vi "V-Meter Shutdown (3706).vi"(8 "error in (no error)":errorcluster, 11 "VISA resource name in":refnum<visa-resource-name>) -> (0 "error out":errorcluster, 3 "VISA resource name out":refnum<visa-resource-name>)   [LabVIEW 2016, in "Hall Effect Library.lvlib"]
uses:
  Hall Effect Library.lvlib
  <instrlib>/Keithley 3706/Keithley 3706.lvlib
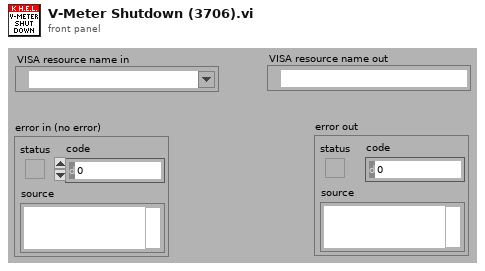
[diagram p1: front panel]
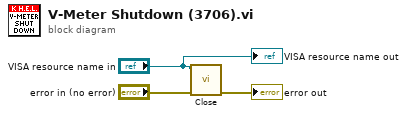
[diagram p0: block diagram]
diagram:
  n1 = call <instrlib>:"Close.vi"("error in (no error)"="error in (no error)", "VISA resource name"="VISA resource name in") -> ("error out"=→"error out":errorcluster)  [unwired: 9 in]
  "VISA resource name out" <- "VISA resource name in"
